vi "Select plot.vi"(6 "Coords":T1, 8 "error in (no error)":errorcluster, 11 "Waveform Ref":T2) -> (0 "error out":errorcluster, 1 "Do not update":bool, 2 "Plot Number":i32)   [LabVIEW 2017, in "XGrapher.xctl"]
uses:
  XGrapher.xctl
  Typedefs/Xctrl-Timeline graph ref.ctl
  <vilib>/Utility/miscctls.llb/LVPoint32TypeDef.ctl
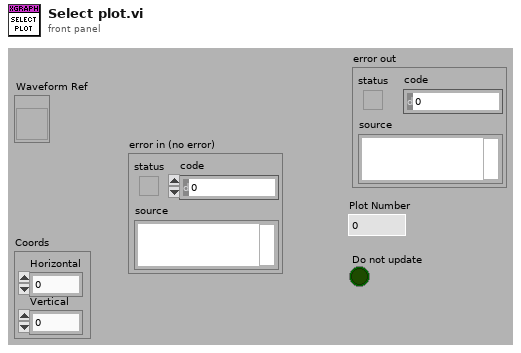
[diagram p1: front panel]
types:
  T1 = typedef "LVPoint32TypeDef.ctl" = cluster{"Horizontal":i32, "Vertical":i32}
  T2 = typedef "XGrapher.xctl/Xctrl-Timeline graph ref.ctl" = refnum<vi>
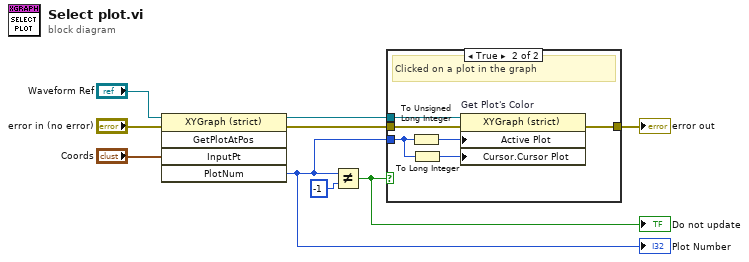
[diagram p0: block diagram]
diagram:
  n1 = invoke on="Invoke Node" class="XYGraph (strict)" method="GetPlotAtPos"(reference="Waveform Ref", error in="error in (no error)", "InputPt"="Coords") -> (reference out=w7:T2, error out=w8:errorcluster, "PlotNum"=w1:i32)  [unwired: 2 in, 2 out]
  "Plot Number" <- w1
  n2 = Not Equal?(x=w1, y=-1) -> (x != y?=w2:bool)
  "Do not update" <- w2
  n3 = case shown="True" w2 {
    tunnel: w8 -> [w10 w16]
    tunnel: w7 -> [_ w15]
    tunnel: w1 -> [_ w12]
    tunnel: [w10 w14] -> w3
    frame False {
      # "Clicked elsewhere on the graph"
    }
    frame True {
      # "Clicked on a plot in the graph"
      n4 = To Unsigned Long Integer(number=w12) -> (unsigned 32bit integer=w13:u32)
      n5 = To Long Integer(number=w12) -> (32bit integer=w11:i32)
      n6 = property on="Get Plot's Color" class="XYGraph (strict)"(reference=w15, error in=w16, "Active Plot"=w13, "Cursor.Cursor Plot"=w11) -> (error out=w14:errorcluster)  [unwired: 1 out]
    }
  }
  "error out" <- w3
